vi "OO_Spectra.vi"() -> ()   [LabVIEW 2016, in "Pressure Gage.lvclass"]
uses:
  Pressure Gage.lvclass
  Utilities/Fit/Multi-peak Parameters.ctl
  Utilities/Fit/Peak Parameters.ctl
  Pressure Gage.lvclass/Pressure Gage.ctl
  File/Controls/File formats.ctl
  <instrlib>/Ocean Optics 2000 4000/Ocean Optics 2000 4000.lvlib
panel:
  in  "Fit avg":bool
  in  "Follow peak":bool
  in  "Background":path=path "C:/Data/February_2018/021618/pspec003_021618.tdms"
  out "# of spectra":i32
  in  "Stop Button":bool
  in  "Fit parameters":T1={"Function"=enum."Lorentz", "Window width"=1.0, "Initial guess"={"Amplitude"=1000.0, "Center"=694.3, "Width"=0.4}} {"Initial guess"."Width" format="%#_gnm"; "Initial guess"."Center" format="%#_gnm"; "Window width" format="%#_6gnm"}
  out "Chart file":path
  in  "Save chart":bool
  out "Spectrum file":path
  in  "Save spectrum":bool
  in  "Integration time":dbl=0.5 format="%#_6ps"
  out "Pressure":dbl(graph)=7.520465813546207
  in  "Reference wavelengh":dbl=694.123
  out "Pressure, kBar":dbl=7.520465813546207 format="%#_4g"
  out "Fit result":T1={"Function"=enum."Lorentz", "Window width"=-1.0993239942180182, "Initial guess"={"Amplitude"=1000.0, "Center"=694.3, "Width"=0.4}} {"Initial guess"."Width" format="%#_gnm"; "Initial guess"."Center" format="%#_gnm"; "Window width" format="%#_6gnm"}
  in  "Fit":bool
  out "Spectral Waveform":T3(graph)
  in  "Enable Strobe (Disabled)":bool
  in  "VISA resource name":refnum<visa-resource-name>="MayaPro"
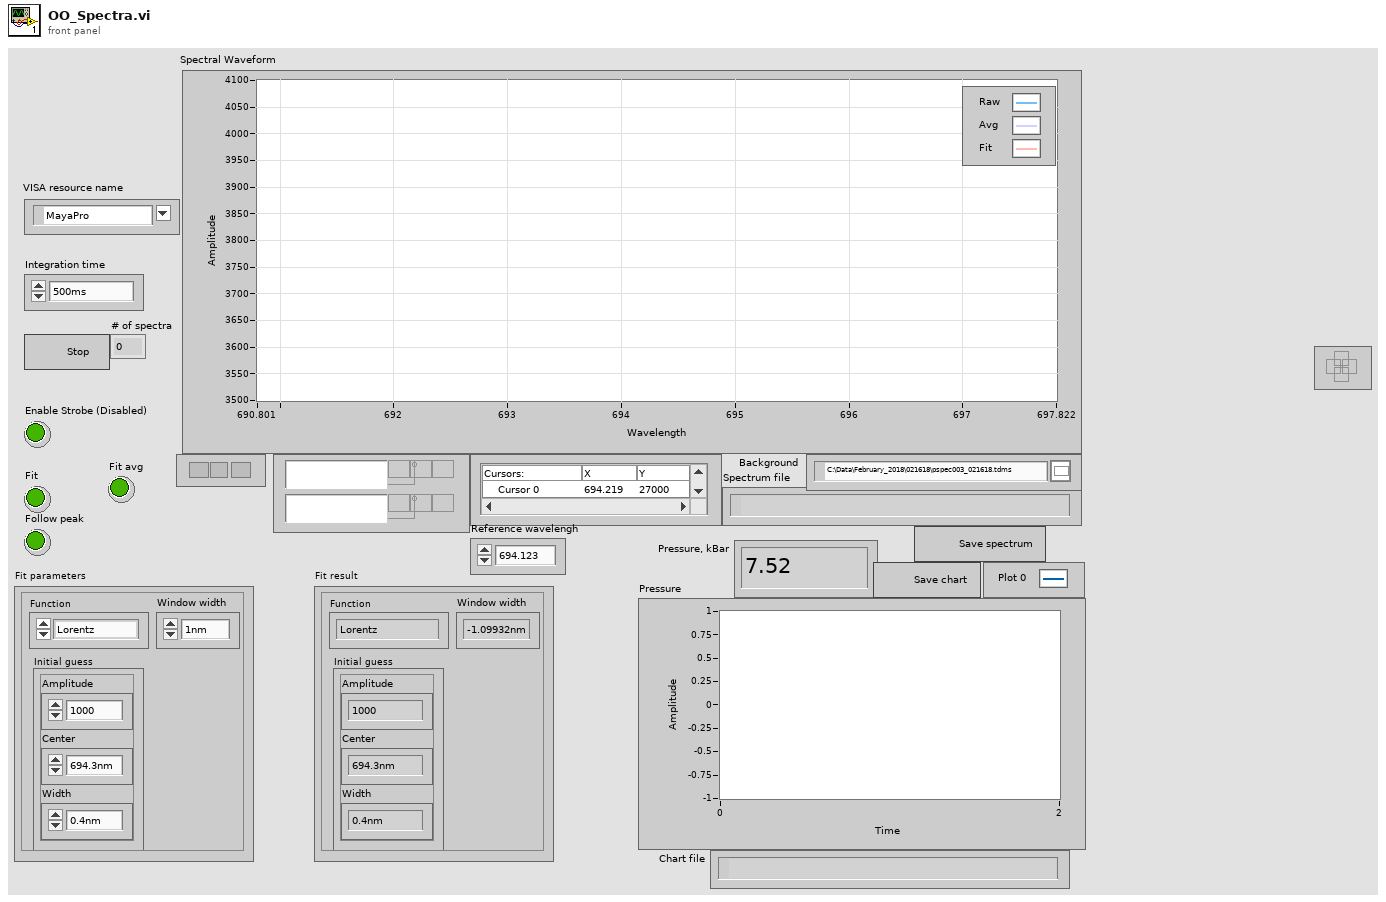
[diagram p1: front panel]
types:
  T1 = typedef "Multi-peak Parameters.ctl" = cluster{"Function":enum16{"Gauss", "Lorentz"}, "Window width":dbl, "Initial guess":T2}
  T2 = typedef "Peak Parameters.ctl" = cluster{"Amplitude":dbl, "Center":dbl, "Width":dbl}
  T3 = cluster{"Wavelength (nm)":dbl[], "Spectrum by Pixel Number":dbl[]}[]
  T4 = typedef "File formats.ctl" = enum16{"TDMS", "ASCII", "BINARY"}
  T5 = enum16{"open", "open or create", "create or replace", "create", "open (read-only)"}
  T6 = cluster{"Wavelengths (nm)":dbl[], "Spectrum out":dbl[]}
  T7 = cluster{"Wavelengths (nm)":dbl[], "Spectrum out":dbl[]}[]
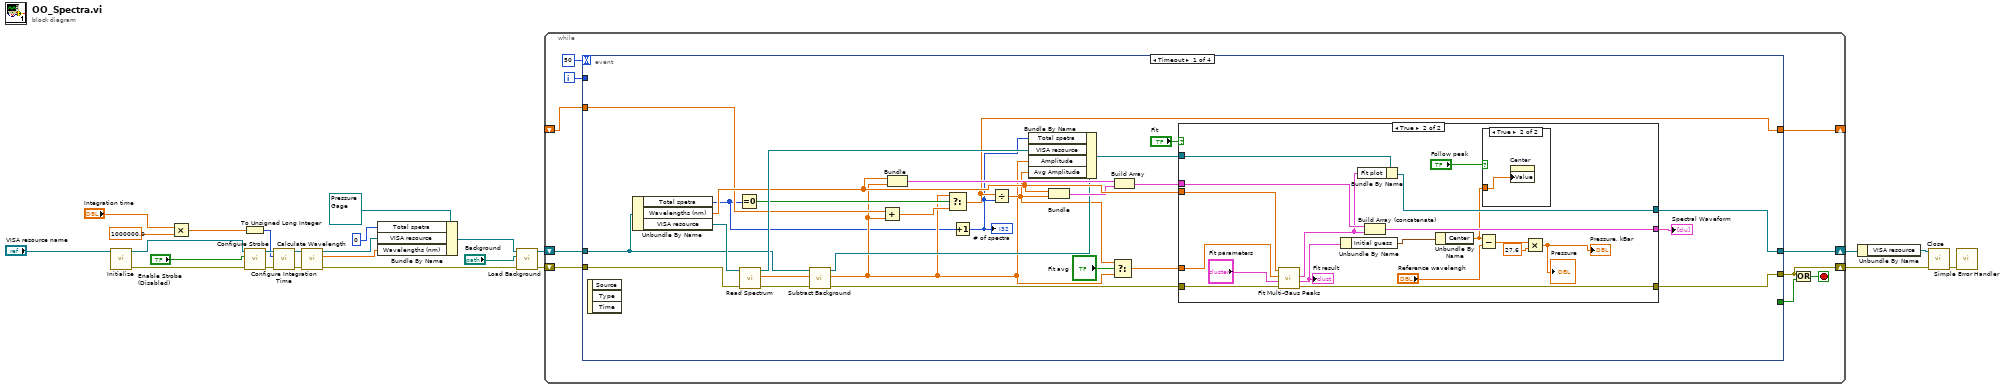
[diagram p0: block diagram]
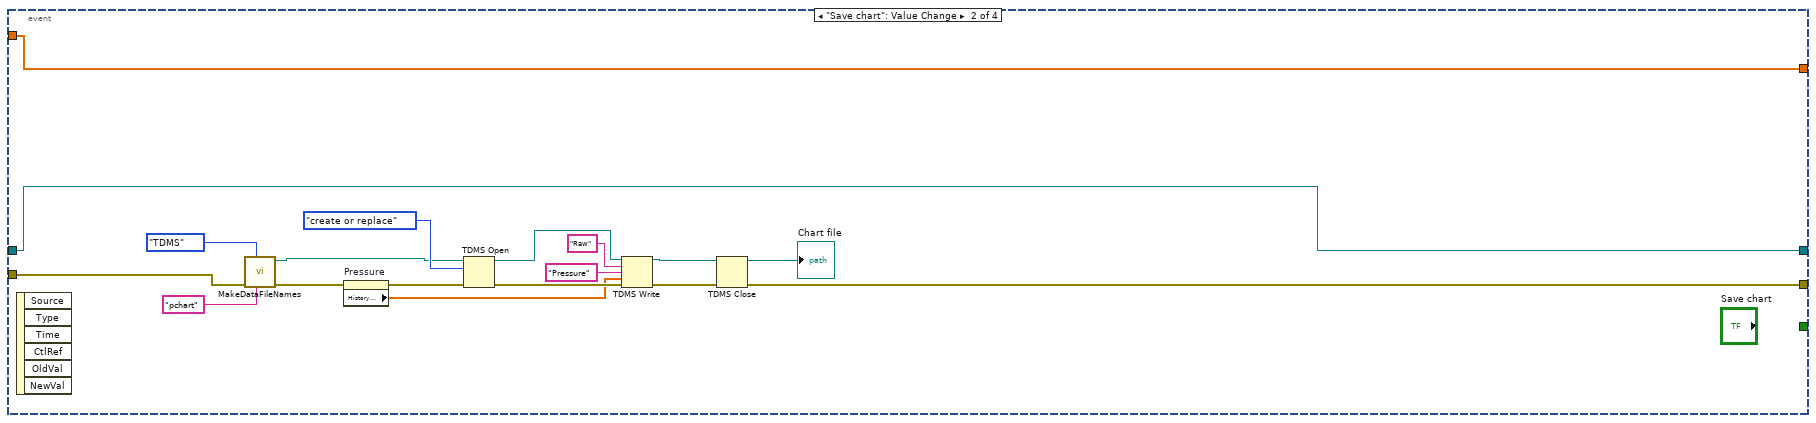
[diagram p4: hidden frame]
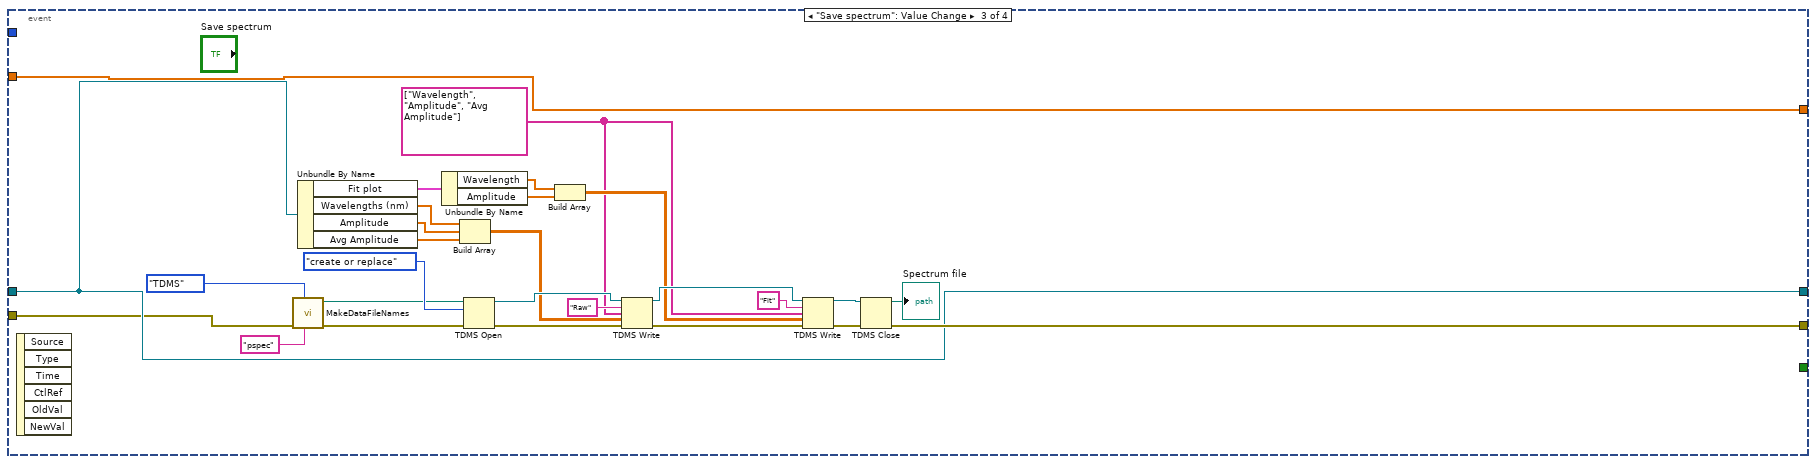
[diagram p5: hidden frame]
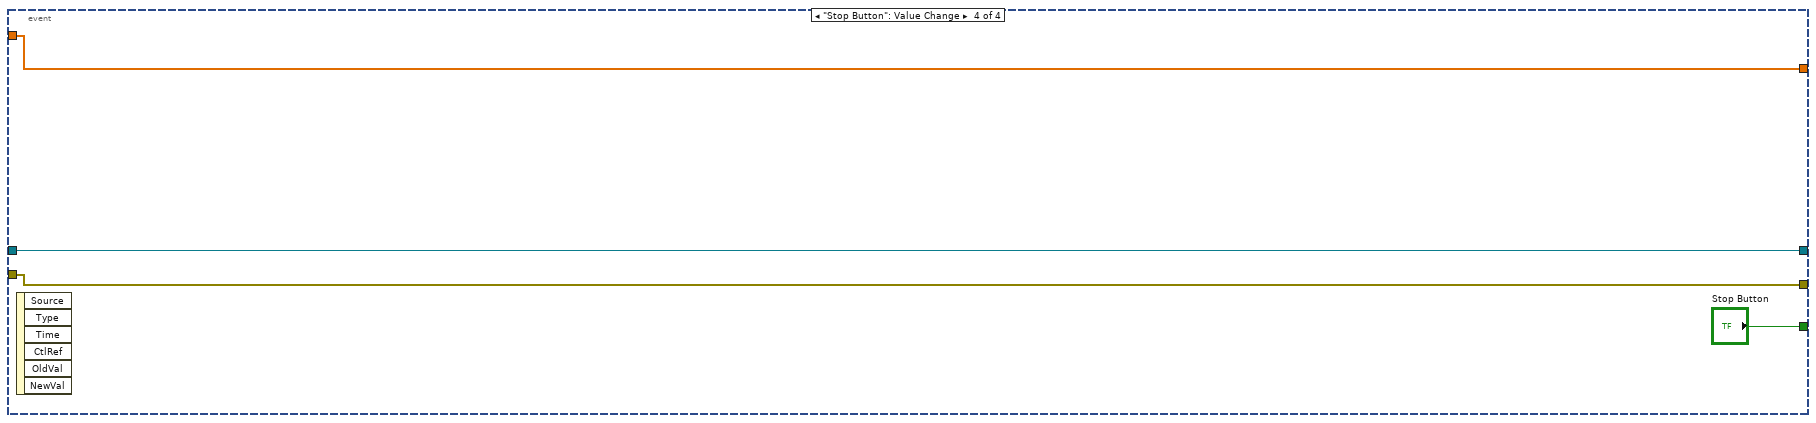
[diagram p6: hidden frame]
diagram:
  n1 = call <instrlib>:"Initialize.vi"("VISA resource name"="VISA resource name") -> ("error out"=w24:errorcluster, "VISA resource name out"=w25:refnum<visa-resource-name>)  [unwired: 2 in, 7 out]
  n2 = Multiply(x="Integration time", y=1000000.0) -> (x*y=w14:dbl)
  n3 = To Unsigned Long Integer(number=w14) -> (unsigned 32bit integer=w13:u32)
  n4 = call <instrlib>:"Configure Strobe.vi"("error in (no error)"=w24, "Enable Strobe (Disabled)"="Enable Strobe (Disabled)", "VISA resource name"=w25) -> ("error out"=w19:errorcluster, "VISA resource name out"=w20:refnum<visa-resource-name>)  [unwired: 7 out]
  n5 = call <instrlib>:"Configure Integration Time.vi"("error in (no error)"=w19, "Integration Time (6000)"=w13, "VISA resource name"=w20) -> ("error out"=w18:errorcluster, "VISA resource name out"=w17:refnum<visa-resource-name>)  [unwired: 7 in]
  n6 = call <instrlib>:"Calculate Wavelength.vi"("error in (no error)"=w18, "VISA resource name"=w17) -> ("error out"=w4:errorcluster, "Wavelength (nm)"=w10:dbl[], "VISA resource name out"=w11:refnum<visa-resource-name>)  [unwired: 1 in, 6 out]
  n7 = Bundle By Name(cluster=refnum<class "Pressure Gage.lvclass"> refnum ("Pressure Gage.lvclass"), "Total spetra"=0, "VISA resource"=w11, "Wavelengths (nm)"=w10) -> (w6:refnum<class "Pressure Gage.lvclass">)
  n8 = call-dynamic "Load Background.vi"("error in (no error)"=w4, "Background"="Background", "Pressure Gage in"=w6) -> ("error out"=w3:errorcluster, "Pressure Gage out"=w5:refnum<class "Pressure Gage.lvclass">)  [unwired: 7 in]
  n9 = while {
    shift-right: [w33] -> w23
    shift-left: w3 -> [w35]
    shift-right: [w29] -> w9
    shift-left: w5 -> [w30]
    shift-right: [w28] -> _
    shift-left: _ -> [w27]
    i -> [w26]
    stop <- w34 stop-if-true
    n10 = event shown="[0] Timeout" {
      selector: _ -> [_ _ _ _]
      dyn-events: _ -> [_ _ _ _]
      timeout: 50 -> [_ _ _ _]
      tunnel: w35 -> [w62 w90 w108 w133]
      tunnel: [w55 w92 w114 w133] -> w33
      tunnel: [_ _ _ "Stop Button"] -> w31
      tunnel: w30 -> [w46 w91 w111 w132]
      tunnel: [w56 w91 w111 w132] -> w29
      tunnel: w26 -> [_ _ _ _]
      tunnel: [w47 w85 w103 w130] -> w28
      tunnel: w27 -> [w48 w85 w103 w130]
      event Timeout {
        n11 = event-data() -> ()  [unwired: 1 in, 3 out]
        n12 = Unbundle By Name(w46) -> ("Total spetra"=w37:i32, "Wavelengths (nm)"=w50:dbl[], "VISA resource"=w59:refnum<visa-resource-name>)
        n13 = Equal To 0?(x=w37) -> (x = 0?=w54:bool)
        n14 = call <instrlib>:"Read Spectrum.vi"("error in (no error)"=w62, "VISA resource name"=w59) -> ("error out"=w43:errorcluster, "Spectrum by Pixel Number"=w44:dbl[], "VISA resource name out"=w58:refnum<visa-resource-name>)  [unwired: 6 in, 1 out]
        n15 = call-dynamic "Subtract Background.vi"("error in (no error)"=w43, "Spectrum"=w44, "Pressure Gage in"=w46) -> ("error out"=w42:errorcluster, "Spectrum out"=w39:dbl[], "Pressure Gage out"=w45:refnum<class "Pressure Gage.lvclass">)  [unwired: 6 in]
        n16 = Add(x=w48, y=w39) -> (x+y=w53:dbl[])
        n17 = Bundle("Wavelengths (nm)"=w50, "Spectrum out"=w39) -> (w52:T6)  [unwired: 1 out]
        n18 = Select(t=w39, s=w54, f=w53) -> (s? t:f=w47:dbl[])
        n19 = Increment(x=w37) -> (x+1=w36:i32)
        "# of spectra" <- w36
        n20 = Divide(x=w47, y=w36) -> (x/y=w40:dbl[])
        n21 = Bundle By Name(cluster=w45, "Total spetra"=w36, "VISA resource"=w58, "Amplitude"=w39, "Avg Amplitude"=w40) -> (w57:refnum<class "Pressure Gage.lvclass">)
        n22 = Bundle("Wavelengths (nm)"=w50, w40) -> (w49:cluster{"Wavelengths (nm)":dbl[], dbl[]})  [unwired: 1 out]
        n23 = Select(t=w40, s="Fit avg", f=w39) -> (s? t:f=w38:dbl[])
        n24 = Build Array(w52, w49) -> (w51:T7)
        n25 = case shown="True" "Fit" {
          tunnel: w50 -> [_ w83]
          tunnel: w38 -> [_ w82]
          tunnel: w51 -> [w65 w81]
          tunnel: [w65 w80] -> w60
          tunnel: w57 -> [w64 w74]
          tunnel: [w64 w72] -> w56
          tunnel: w42 -> [w63 w70]
          tunnel: [w63 w69] -> w55
          frame False {
          }
          frame True {
            n26 = call "Fit Multi-Gaus Peaks.vi"("Error In"=w70, "Fit parameters"="Fit parameters", "Y"=w82, "X"=w83) -> ("Error Out"=w69:errorcluster, "Fit parameters out"=w79:T1, "Fit plot"=w73:cluster{"Array":dbl[], "Array":dbl[]})  [unwired: 5 in]
            "Fit result" <- w79
            n27 = Unbundle By Name(w79) -> ("Initial guess"=w66:T2)
            n28 = Bundle By Name(cluster=w74, "Fit plot"=w73) -> (w72:refnum<class "Pressure Gage.lvclass">)
            n29 = Build Array (concatenate)(w81, w73) -> (w80:cluster{"Array":dbl[], "Array":dbl[]}[])
            n30 = Unbundle By Name(w66) -> ("Center"=w67:dbl)
            n31 = Subtract(x=w67, y="Reference wavelengh") -> (x-y=w77:dbl)
            n32 = case shown="True" "Follow peak" {
              tunnel: w67 -> [_ w84]
              frame False {
              }
              frame True {
                n33 = property on="Center" class="DigNum (strict)"("Value"=w84) -> ()  [unwired: 2 in, 2 out]
              }
            }
            n34 = Multiply(x=w77, y=27.6) -> (x*y=→"Pressure, kBar" →"Pressure":dbl)
          }
        }
        "Spectral Waveform" <- w60
      }
      event "Save chart": Value Change {
        n35 = event-data() -> ()  [unwired: 1 in, 6 out]
        n36 = call "MakeDataFileNames.vi"("File Prefix"="pchart", "File format"=File_formats."TDMS", "Error In"=w90) -> ("Error Out"=w89:errorcluster, "Data File  Path"=w87:path)  [unwired: 5 in, 2 out]
        n37 = property on="Pressure" class="WFChart (strict)"(error in=w89) -> (error out=w95:errorcluster, "History Data"=w94:dbl[])  [unwired: 1 in, 1 out]
        n38 = TDMS Open(8:w95, 10:T5."create or replace" ("operation (0:open)"), 11:w87) -> (0:w101:errorcluster, 3:w100:refnum<k34>)  [unwired: 4 in]
        n39 = TDMS Write(0:w100, 5:"Raw" ("group name in (Untitled)"), 7:"Pressure", 9:w94, 11:w101) -> (4:w98:refnum<k34>, 15:w97:errorcluster)  [unwired: 1 in, 2 out]
        n40 = TDMS Close(8:w97, 11:w98) -> (0:w92:errorcluster, 3:→"Chart file":path)
      }
      event "Save spectrum": Value Change {
        w117 = string[] ["Wavelength", "Amplitude", "Avg Amplitude"]
        n41 = event-data() -> ()  [unwired: 1 in, 6 out]
        n42 = call "MakeDataFileNames.vi"("File Prefix"="pspec", "File format"=File_formats."TDMS", "Error In"=w108) -> ("Error Out"=w107:errorcluster, "Data File  Path"=w106:path)  [unwired: 5 in, 2 out]
        n43 = Unbundle By Name(w111) -> ("Fit plot"=w121:cluster{"Wavelength":dbl[], "Amplitude":dbl[]}, "Wavelengths (nm)"=w123:dbl[], "Amplitude"=w105:dbl[], "Avg Amplitude"=w104:dbl[])
        n44 = Unbundle By Name(w121) -> ("Wavelength"=w120:dbl[], "Amplitude"=w119:dbl[])
        n45 = Build Array(w123, w105, w104) -> (w122:dbl[][])
        n46 = TDMS Open(8:w107, 10:T5."create or replace" ("operation (0:open)"), 11:w106) -> (0:w128:errorcluster, 3:w127:refnum<k34>)  [unwired: 4 in]
        n47 = Build Array(w120, w119) -> (w118:dbl[][])
        n48 = TDMS Write(0:w127, 5:"Raw" ("group name in (Untitled)"), 7:w117, 9:w122, 11:w128) -> (4:w125:refnum<k34>, 15:w124:errorcluster)  [unwired: 1 in, 2 out]
        n49 = TDMS Write(0:w125, 5:"Fit" ("group name in (Untitled)"), 7:w117, 9:w118, 11:w124) -> (4:w113:refnum<k34>, 15:w115:errorcluster)  [unwired: 1 in, 2 out]
        n50 = TDMS Close(8:w115, 11:w113) -> (0:w114:errorcluster, 3:→"Spectrum file":path)
      }
      event "Stop Button": Value Change {
        n51 = event-data() -> ()  [unwired: 1 in, 6 out]
      }
    }
    n52 = Or(x=w33, y=w31) -> (x .or. y?=w34:bool)
  }
  n53 = Unbundle By Name(w9) -> ("VISA resource"=w8:refnum<visa-resource-name>)
  n54 = call <instrlib>:"Close.vi"("error in (no error)"=w23, "VISA resource name"=w8) -> ("error out"=w22:errorcluster)  [unwired: 9 out]
  n55 = call <vilib>:"Simple Error Handler.vi"("error in (no error)"=w22) -> ()  [unwired: 1 in, 8 out]
